vi "Setproperty_id.vi"(8 "error in (no error)":errorcluster, 10 "Set_Val":T1, 11 "OneOfTemplate in":refnum<class "nixnet_grpc_DbGetPropertySizeRequest_property_id_enum.lvclass">) -> (0 "error out":errorcluster, 3 "OneOfTemplate out":refnum<class "nixnet_grpc_DbGetPropertySizeRequest_property_id_enum.lvclass">)   [LabVIEW 2019, in "grpc-xnet_client.lvlib" / "nixnet_grpc_DbGetPropertySizeRequest_property_id_enum.lvclass"]
uses:
  nixnet_grpc_DbGetPropertySizeRequest_property_id_enum.lvclass
  nixnet_grpc_DBProperty.ctl
  nixnet_grpc_DbGetPropertySizeRequest_property_id_enum.lvclass/nixnet_grpc_DbGetPropertySizeRequest_property_id_enum.ctl
  grpc-xnet_client.lvlib
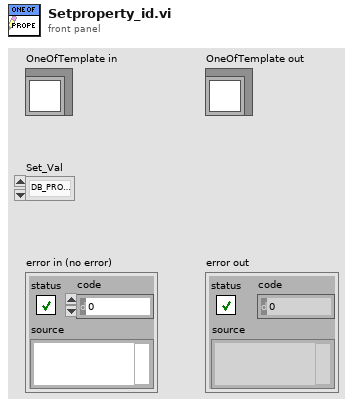
[diagram p1: front panel]
types:
  T1 = typedef "grpc-xnet_client.lvlib/nixnet_grpc_DBProperty.ctl" = enum32{"DB_PROPERTY_UNSPECIFIED", "DB_PROPERTY_DATABASE_CLST_REFS", "DB_PROPERTY_DATABASE_NAME", "DB_PROPERTY_DATABASE_SHOW_INVALID_FROM_OPEN", "DB_PROPERTY_CLST_BAUD_RATE_64", "DB_PROPERTY_CLST_APPLICATION_PROTOCOL", "DB_PROPERTY_CLST_BAUD_RATE", "DB_PROPERTY_CLST_CAN_FD_BAUD_RATE_64", "DB_PROPERTY_CLST_CAN_FD_BAUD_RATE", "DB_PROPERTY_CLST_CAN_FD_ISO_MODE", "DB_PROPERTY_CLST_CAN_IO_MODE", "DB_PROPERTY_CLST_COMMENT", "DB_PROPERTY_CLST_CONFIG_STATUS", "DB_PROPERTY_CLST_DATABASE_REF", "DB_PROPERTY_CLST_ECU_REFS", "DB_PROPERTY_CLST_FLEX_RAY_ACT_PT_OFF", "DB_PROPERTY_CLST_FLEX_RAY_ALW_PASS_ACT", "DB_PROPERTY_CLST_FLEX_RAY_CAS_RX_L_MAX", "DB_PROPERTY_CLST_FLEX_RAY_CHANNELS", "DB_PROPERTY_CLST_FLEX_RAY_CLST_DRIFT_DMP", "DB_PROPERTY_CLST_FLEX_RAY_COLD_ST_ATS", "DB_PROPERTY_CLST_FLEX_RAY_CYCLE", "DB_PROPERTY_CLST_FLEX_RAY_DYN_SEG_START", "DB_PROPERTY_CLST_FLEX_RAY_DYN_SLOT_IDL_PH", "DB_PROPERTY_CLST_FLEX_RAY_LATEST_GUAR_DYN", "DB_PROPERTY_CLST_FLEX_RAY_LATEST_USABLE_DYN", "DB_PROPERTY_CLST_FLEX_RAY_LIS_NOISE", "DB_PROPERTY_CLST_FLEX_RAY_MACRO_PER_CYCLE", "DB_PROPERTY_CLST_FLEX_RAY_MACROTICK", "DB_PROPERTY_CLST_FLEX_RAY_MAX_WO_CLK_COR_FAT", "DB_PROPERTY_CLST_FLEX_RAY_MAX_WO_CLK_COR_PAS", "DB_PROPERTY_CLST_FLEX_RAY_MINISLOT", "DB_PROPERTY_CLST_FLEX_RAY_MINISLOT_ACT_PT", "DB_PROPERTY_CLST_FLEX_RAY_NIT", "DB_PROPERTY_CLST_FLEX_RAY_NIT_START", "DB_PROPERTY_CLST_FLEX_RAY_NM_VEC_LEN", "DB_PROPERTY_CLST_FLEX_RAY_NUM_MINISLT", "DB_PROPERTY_CLST_FLEX_RAY_NUM_STAT_SLT", "DB_PROPERTY_CLST_FLEX_RAY_OFF_COR_ST", "DB_PROPERTY_CLST_FLEX_RAY_PAYLD_LEN_DYN_MAX", "DB_PROPERTY_CLST_FLEX_RAY_PAYLD_LEN_MAX", "DB_PROPERTY_CLST_FLEX_RAY_PAYLD_LEN_ST", "DB_PROPERTY_CLST_FLEX_RAY_STAT_SLOT", "DB_PROPERTY_CLST_FLEX_RAY_SYM_WIN", "DB_PROPERTY_CLST_FLEX_RAY_SYM_WIN_START", "DB_PROPERTY_CLST_FLEX_RAY_SYNC_NODE_MAX", "DB_PROPERTY_CLST_FLEX_RAY_TSS_TX", "DB_PROPERTY_CLST_FLEX_RAY_USE_WAKEUP", "DB_PROPERTY_CLST_FLEX_RAY_WAKE_SYM_RX_IDL", "DB_PROPERTY_CLST_FLEX_RAY_WAKE_SYM_RX_LOW", "DB_PROPERTY_CLST_FLEX_RAY_WAKE_SYM_RX_WIN", "DB_PROPERTY_CLST_FLEX_RAY_WAKE_SYM_TX_IDL", "DB_PROPERTY_CLST_FLEX_RAY_WAKE_SYM_TX_LOW", "DB_PROPERTY_CLST_FRM_REFS", "DB_PROPERTY_CLST_LIN_SCHEDULES", "DB_PROPERTY_CLST_LIN_TICK", "DB_PROPERTY_CLST_NAME", "DB_PROPERTY_CLST_PDU_REFS", "DB_PROPERTY_CLST_PD_US_REQD", "DB_PROPERTY_CLST_PROTOCOL", "DB_PROPERTY_CLST_SIG_REFS", "DB_PROPERTY_FRM_APPLICATION_PROTOCOL", "DB_PROPERTY_FRM_CAN_EXT_ID", "DB_PROPERTY_FRM_CAN_IO_MODE", "DB_PROPERTY_FRM_CAN_TIMING_TYPE", "DB_PROPERTY_FRM_CAN_TX_TIME", "DB_PROPERTY_FRM_CLUSTER_REF", "DB_PROPERTY_FRM_COMMENT", "DB_PROPERTY_FRM_CONFIG_STATUS", "DB_PROPERTY_FRM_DEFAULT_PAYLOAD", "DB_PROPERTY_FRM_FLEX_RAY_BASE_CYCLE", "DB_PROPERTY_FRM_FLEX_RAY_CH_ASSIGN", "DB_PROPERTY_FRM_FLEX_RAY_CYCLE_REP", "DB_PROPERTY_FRM_FLEX_RAY_IN_CYC_REP_CH_ASSIGNS", "DB_PROPERTY_FRM_FLEX_RAY_IN_CYC_REP_ENABLED", "DB_PROPERTY_FRM_FLEX_RAY_IN_CYC_REP_IDS", "DB_PROPERTY_FRM_FLEX_RAY_PREAMBLE", "DB_PROPERTY_FRM_FLEX_RAY_STARTUP", "DB_PROPERTY_FRM_FLEX_RAY_SYNC", "DB_PROPERTY_FRM_FLEX_RAY_TIMING_TYPE", "DB_PROPERTY_FRM_ID", "DB_PROPERTY_FRM_LIN_CHECKSUM", "DB_PROPERTY_FRM_MUX_DATA_MUX_SIG_REF", "DB_PROPERTY_FRM_MUX_IS_MUXED", "DB_PROPERTY_FRM_MUX_STATIC_SIG_REFS", "DB_PROPERTY_FRM_MUX_SUBFRAME_REFS", "DB_PROPERTY_FRM_NAME", "DB_PROPERTY_FRM_PDU_START_BITS", "DB_PROPERTY_FRM_PDU_UPDATE_BITS", "DB_PROPERTY_FRM_PDU_REFS", "DB_PROPERTY_FRM_PAYLOAD_LEN", "DB_PROPERTY_FRM_SIG_REFS", "DB_PROPERTY_FRM_VARIABLE_PAYLOAD", "DB_PROPERTY_SIG_BYTE_ORDR", "DB_PROPERTY_SIG_COMMENT", "DB_PROPERTY_SIG_CONFIG_STATUS", "DB_PROPERTY_SIG_DATA_TYPE", "DB_PROPERTY_SIG_DEFAULT", "DB_PROPERTY_SIG_FRAME_REF", "DB_PROPERTY_SIG_MAX", "DB_PROPERTY_SIG_MIN", "DB_PROPERTY_SIG_MUX_IS_DATA_MUX", "DB_PROPERTY_SIG_MUX_IS_DYNAMIC", "DB_PROPERTY_SIG_MUX_VALUE", "DB_PROPERTY_SIG_MUX_SUBFRM_REF", "DB_PROPERTY_SIG_NAME", "DB_PROPERTY_SIG_NAME_UNIQUE_TO_CLUSTER", "DB_PROPERTY_SIG_NUM_BITS", "DB_PROPERTY_SIG_PDU_REF", "DB_PROPERTY_SIG_SCALE_FAC", "DB_PROPERTY_SIG_SCALE_OFF", "DB_PROPERTY_SIG_START_BIT", "DB_PROPERTY_SIG_UNIT", "DB_PROPERTY_SUBFRM_CONFIG_STATUS", "DB_PROPERTY_SUBFRM_DYN_SIG_REFS", "DB_PROPERTY_SUBFRM_FRM_REF", "DB_PROPERTY_SUBFRM_MUX_VALUE", "DB_PROPERTY_SUBFRM_NAME", "DB_PROPERTY_SUBFRM_NAME_UNIQUE_TO_CLUSTER", "DB_PROPERTY_SUBFRM_PDU_REF", "DB_PROPERTY_ECU_CLST_REF", "DB_PROPERTY_ECU_COMMENT", "DB_PROPERTY_ECU_CONFIG_STATUS", "DB_PROPERTY_ECU_FLEX_RAY_IS_COLDSTART", "DB_PROPERTY_ECU_FLEX_RAY_CONNECTED_CHS", "DB_PROPERTY_ECU_FLEX_RAY_STARTUP_FRAME_REF", "DB_PROPERTY_ECU_FLEX_RAY_WAKEUP_CHS", "DB_PROPERTY_ECU_FLEX_RAY_WAKEUP_PTRN", "DB_PROPERTY_ECU_RX_FRM_REFS", "DB_PROPERTY_ECU_TX_FRM_REFS", "DB_PROPERTY_ECU_LIN_CONFIG_NAD", "DB_PROPERTY_ECU_LIN_FUNCTION_ID", "DB_PROPERTY_ECU_LIN_INITIAL_NAD", "DB_PROPERTY_ECU_LIN_MASTER", "DB_PROPERTY_ECU_LINP2MIN", "DB_PROPERTY_ECU_LIN_PROTOCOL_VER", "DB_PROPERTY_ECU_LINS_TMIN", "DB_PROPERTY_ECU_LIN_SUPPLIER_ID", "DB_PROPERTY_ECU_NAME", "DB_PROPERTY_ECU_J1939_NODE_NAME", "DB_PROPERTY_ECU_J1939_PREFERRED_ADDRESS", "DB_PROPERTY_LIN_SCHED_CLST_REF", "DB_PROPERTY_LIN_SCHED_COMMENT", "DB_PROPERTY_LIN_SCHED_CONFIG_STATUS", "DB_PROPERTY_LIN_SCHED_ENTRIES", "DB_PROPERTY_LIN_SCHED_NAME", "DB_PROPERTY_LIN_SCHED_PRIORITY", "DB_PROPERTY_LIN_SCHED_RUN_MODE", "DB_PROPERTY_LIN_SCHED_ENTRY_COLLISION_RES_SCHED", "DB_PROPERTY_LIN_SCHED_ENTRY_DELAY", "DB_PROPERTY_LIN_SCHED_ENTRY_EVENT_ID", "DB_PROPERTY_LIN_SCHED_ENTRY_FRAMES", "DB_PROPERTY_LIN_SCHED_ENTRY_NAME", "DB_PROPERTY_LIN_SCHED_ENTRY_NAME_UNIQUE_TO_CLUSTER", "DB_PROPERTY_LIN_SCHED_ENTRY_NC_FF_DATA_BYTES", "DB_PROPERTY_LIN_SCHED_ENTRY_SCHED", "DB_PROPERTY_LIN_SCHED_ENTRY_TYPE", "DB_PROPERTY_PDU_CLUSTER_REF", "DB_PROPERTY_PDU_COMMENT", "DB_PROPERTY_PDU_CONFIG_STATUS", "DB_PROPERTY_PDU_DEFAULT_PAYLOAD", "DB_PROPERTY_PDU_FRM_REFS", "DB_PROPERTY_PDU_MUX_DATA_MUX_SIG_REF", "DB_PROPERTY_PDU_MUX_IS_MUXED", "DB_PROPERTY_PDU_MUX_STATIC_SIG_REFS", "DB_PROPERTY_PDU_MUX_SUBFRAME_REFS", "DB_PROPERTY_PDU_NAME", "DB_PROPERTY_PDU_PAYLOAD_LEN", "DB_PROPERTY_PDU_SIG_REFS"}
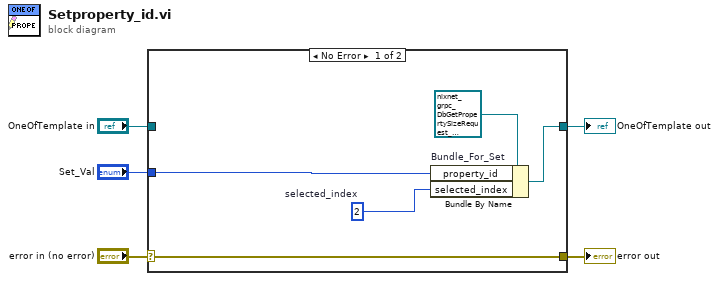
[diagram p0: block diagram]
diagram:
  n1 = case shown="No Error" "error in (no error)" {
    selector: "error in (no error)" -> [w10 w11]
    tunnel: [w10 w11] -> w4
    tunnel: [w9 w12] -> w2
    tunnel: "OneOfTemplate in" -> [_ w12]
    tunnel: "Set_Val" -> [w8 _]
    frame No Error {
      w7 = 2  # selected_index
      n2 = Bundle By Name "Bundle_For_Set"(cluster=refnum<class "nixnet_grpc_DbGetPropertySizeRequest_property_id_enum.lvclass"> refnum ("OneOfTemplate in"), "property_id"=w8, "selected_index"=w7) -> (w9:refnum<class "nixnet_grpc_DbGetPropertySizeRequest_property_id_enum.lvclass">)
    }
    frame Error {
    }
  }
  "error out" <- w4
  "OneOfTemplate out" <- w2
